vi "Init Events.vi"(8 "error in (no error)":errorcluster, 11 "ControlBindingPanel in":refnum<class "ControlBindingPanel.lvclass">) -> (0 "error out":errorcluster, 3 "ControlBindingPanel out":refnum<class "ControlBindingPanel.lvclass">)   [LabVIEW 2020, in "VolatusGUIEditor.lvlib" / "ControlBindingPanel.lvclass"]
uses:
  ControlBindingPanel.lvclass
  ControlBindingPanel.lvclass/ControlBindingPanel.ctl
  Update Control Data.ctl
  lv-tree-tools/Tree Map/Tree Map/Tree Map.lvclass
  Update Tree Data.ctl
  Incoming Events.ctl
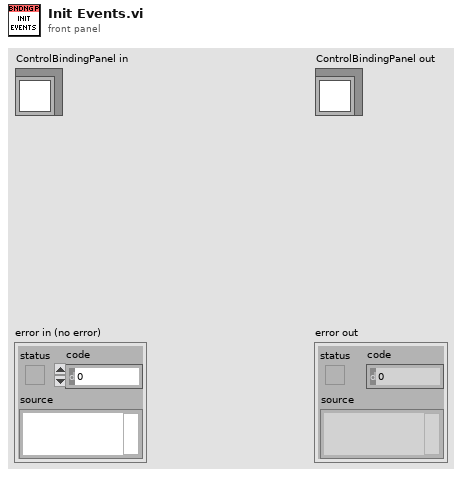
[diagram p1: front panel]
types:
  T1 = typedef "VolatusGUIEditor.lvlib/ControlBindingPanel.lvclass/Incoming Events.ctl" = cluster{"Update Control":refnum<user-event>, "Update Tree":refnum<user-event>}
  T2 = typedef "VolatusGUIEditor.lvlib/ControlBindingPanel.lvclass/Update Tree Data.ctl" = cluster{"Tree Map":refnum<class "Tree Map.lvclass">}
  T3 = typedef "VolatusGUIEditor.lvlib/ControlBindingPanel.lvclass/Update Control Data.ctl" = cluster{"Control":refnum<vi>}
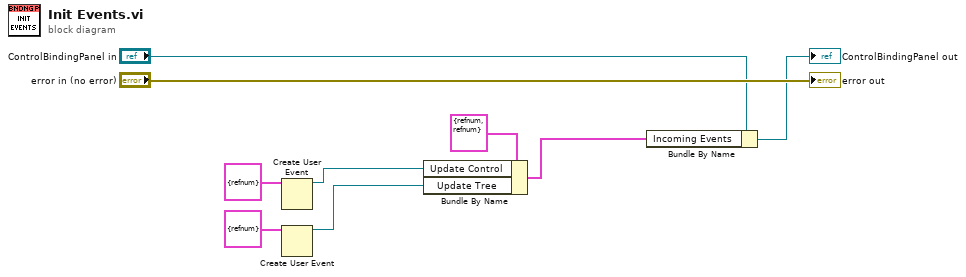
[diagram p0: block diagram]
diagram:
  n1 = Create User Event(user event datatype=T3 {"Control"=refnum} ("Update Control Data")) -> (user event=w4:refnum<user-event>)  [unwired: 1 in, 1 out]
  n2 = Create User Event(user event datatype=T2 {"Tree Map"=refnum} ("Update Tree Data")) -> (user event=w3:refnum<user-event>)  [unwired: 1 in, 1 out]
  n3 = Bundle By Name(cluster=T1 {"Update Control"=refnum, "Update Tree"=refnum} ("Incoming Events"), "Update Control"=w4, "Update Tree"=w3) -> (w2:T1)
  n4 = Bundle By Name(cluster="ControlBindingPanel in", "Incoming Events"=w2) -> (→"ControlBindingPanel out":refnum<class "ControlBindingPanel.lvclass">)
  "error out" <- "error in (no error)"
